vi "8-bit video export-AVI create by mode.vi"(8 "error in (no error)":errorcluster, 11 "8-bit AVI file path":path) -> (0 "error out":errorcluster, 3 "AVI modes refs":T1)   [LabVIEW 2013]
uses:
  Typedefs/8-bit video export AVI modes cluster.ctl
  <vilib>/vision/Avi1.llb/AviRefnum.ctl
  <vilib>/vision/Avi.llb/IMAQ AVI2 Refnum.ctl
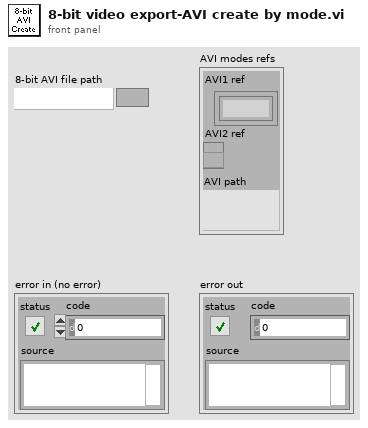
[diagram p1: front panel]
types:
  T1 = typedef "8-bit video export AVI modes cluster.ctl" = cluster{"AVI1 ref":T2, "AVI2 ref":T3, "AVI path":path}
  T2 = typedef "AviRefnum.ctl" = refnum<k1>
  T3 = typedef "IMAQ AVI2 Refnum.ctl" = refnum<k20>
  T4 = typedef "AVI implementation enum.ctl" = enum16{"AVI1", "AVI2"}
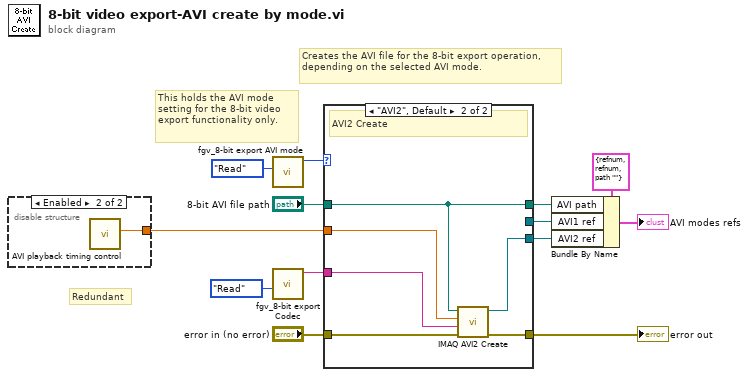
[diagram p0: block diagram]
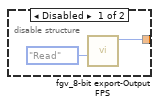
[diagram p2: hidden frame]
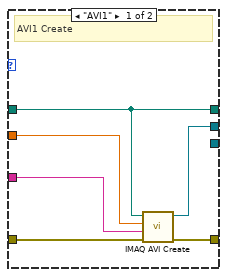
[diagram p3: hidden frame]
diagram:
  # "Redundant"
  # "Creates the AVI file for the 8-bit export operation, depending on the selected AVI mode."
  # "This holds the AVI mode setting for the 8-bit video export functionality only."
  n1 = disable-structure shown="Enabled" {
    disable-tunnel: [w14 w16] -> w1
    frame Disabled {
      n2 = call "fgv_8-bit export-Output FPS.vi"("Function"=enum16{"Intialize", "Write", "Read", "Clear"}."Read") -> ("Frames Per Second"=w14:u32)  [unwired: 9 in, 1 out]
    }
    frame Enabled {
      n3 = call "AVI playback timing control.vi"() -> ("Frame rate set OR original (fps)"=w16:dbl)  [unwired: 8 in, 3 out]
    }
  }
  n4 = call "fgv_8-bit export AVI mode.vi"("Function"=enum16{"Intialize", "Write", "Read", "Clear"}."Read") -> ("AVI mode"=w5:T4)  [unwired: 9 in, 1 out]
  n5 = call "fgv_8-bit export Codec.vi"("Function"=enum16{"Intialize", "Write", "Read", "Clear"}."Read") -> ("AVI mode"=w2:string)  [unwired: 9 in, 1 out]
  n6 = case shown="\"AVI2\", Default" w5 {
    tunnel: "error in (no error)" -> [w22 w26]
    tunnel: [w21 w27] -> w12
    tunnel: w1 -> [w20 w24]
    tunnel: "8-bit AVI file path" -> [w18 w25]
    tunnel: [w19 _] -> w8
    tunnel: [_ w28] -> w7
    tunnel: [w18 w25] -> w4
    tunnel: w2 -> [w17 w23]
    frame "AVI1" {
      # "AVI1 Create"
      n7 = call "IMAQ AVI Create"("error in (no error)"=w22, "Compression Filter"=w17, "Frames Per Second"=w20, "AVI Path"=w18) -> ("error out"=w21:errorcluster, "Avi Refnum"=w19:T2)  [unwired: 6 in]
    }
    frame "AVI2", Default {
      # "AVI2 Create"
      n8 = call "IMAQ AVI2 Create"("error in (no error)"=w26, "Codec"=w23, "Frames Per Second"=w24, "AVI Path"=w25) -> ("error out"=w27:errorcluster, "AVI Refnum"=w28:T3)  [unwired: 6 in]
    }
  }
  "error out" <- w12
  n9 = Bundle By Name(cluster=T1 {"AVI1 ref"=refnum, "AVI2 ref"=refnum, "AVI path"=path ""} ("AVI modes refs"), "AVI path"=w4, "AVI1 ref"=w8, "AVI2 ref"=w7) -> (→"AVI modes refs":T1)
